vi "Get PotRefNum.vi"(8 "error in (no error)":errorcluster, 10 "Side":enum16{"Left", "Right"}(ring), 11 "drive in":refnum<class "drive.lvclass">) -> (0 "error out":errorcluster, 2 "PotDevRef":T1={"DevStatus"={"status"=FALSE, "code"=0, "source"=""}, "Analog Channel"=enum."Invalid", "Invert Output"=FALSE}, 3 "drive out":refnum<class "drive.lvclass">)   [LabVIEW 2015, in "drive.lvclass"]
uses:
  drive.lvclass
  <vilib>/Rock Robotics/WPI/Potentiometer/WPI_PotentiometerDevRef.ctl
  <vilib>/Rock Robotics/SystemInterfaces/AI/FPGA_AIChannel.ctl
  drive.lvclass/drive.ctl
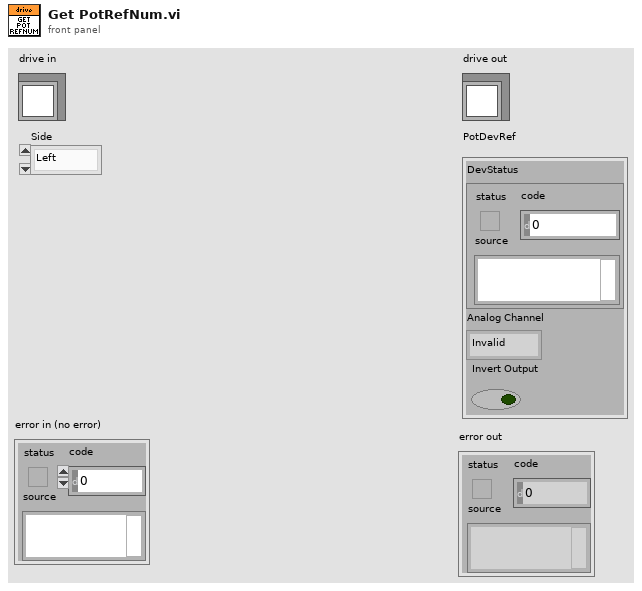
[diagram p1: front panel]
types:
  T1 = typedef "WPI_PotentiometerDevRef.ctl" = cluster{"DevStatus":errorcluster, "Analog Channel":T2, "Invert Output":bool}
  T2 = typedef "FPGA_AIChannel.ctl" = enum8{"AI 0", "AI 1", "AI 2", "AI 3", "AI MXP 0", "AI MXP 1", "AI MXP 2", "AI MXP 3", "Invalid"}
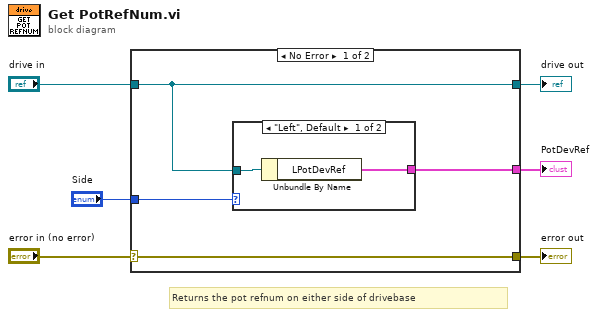
[diagram p0: block diagram]
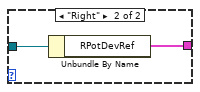
[diagram p2: hidden frame]
diagram:
  # "Returns the pot refnum on either side of drivebase"
  n1 = case shown="No Error" "error in (no error)" {
    selector: "error in (no error)" -> [w10 w15]
    tunnel: [w10 w15] -> w5
    tunnel: [w9 w16] -> w3
    tunnel: "drive in" -> [w9 w16]
    tunnel: [w8 _] -> w2
    tunnel: "Side" -> [w7 _]
    frame No Error {
      n2 = case shown="\"Left\", Default" w7 {
        tunnel: w9 -> [w12 w14]
        tunnel: [w11 w13] -> w8
        frame "Left", Default {
          n3 = Unbundle By Name(w12) -> ("LPotDevRef"=w11:T1)
        }
        frame "Right" {
          n4 = Unbundle By Name(w14) -> ("RPotDevRef"=w13:T1)
        }
      }
    }
    frame Error {
    }
  }
  "error out" <- w5
  "drive out" <- w3
  "PotDevRef" <- w2
